vi "CollectPoint.vi"(8 "error in (no error)":errorcluster, 11 "Snake in":refnum<class "Snake.lvclass">) -> (0 "error out":errorcluster, 3 "Snake out":refnum<class "Snake.lvclass">)   [LabVIEW 2019, in "RT_Game.lvlib" / "Snake.lvclass"]
uses:
  Snake.lvclass
  Snake.lvclass/Snake.ctl
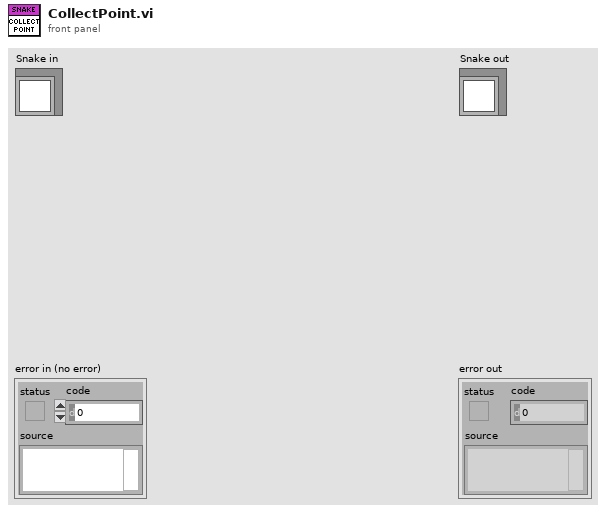
[diagram p1: front panel]
types:
  T1 = typedef "RT_Game.lvlib/Game.lvclass/Coordinate.ctl" = cluster{"x":i16, "y":i16}
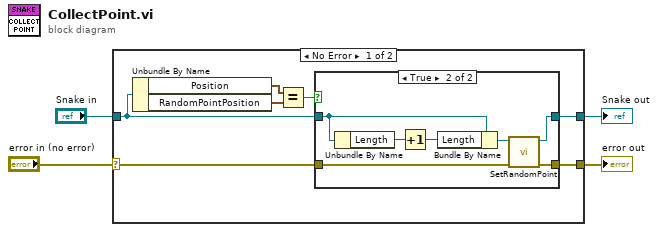
[diagram p0: block diagram]
diagram:
  n1 = case shown="No Error" "error in (no error)" {
    selector: "error in (no error)" -> [w11 w22]
    tunnel: [w8 w22] -> w3
    tunnel: [w7 w21] -> w1
    tunnel: "Snake in" -> [w6 w21]
    frame No Error {
      n2 = Unbundle By Name(w6) -> ("Position"=w9:T1, "RandomPointPosition"=w10:T1)
      n3 = Equal?(x=w9, y=w10) -> (x = y?=w5:bool)
      n4 = case shown="True" w5 {
        tunnel: w11 -> [w12 w20]
        tunnel: [w12 w19] -> w8
        tunnel: [w13 w18] -> w7
        tunnel: w6 -> [w13 w16]
        frame False {
        }
        frame True {
          n5 = Unbundle By Name(w16) -> ("Length"=w15:i16)
          n6 = Increment(x=w15) -> (x+1=w14:i16)
          n7 = Bundle By Name(cluster=w16, "Length"=w14) -> (w17:refnum<class "Snake.lvclass">)
          n8 = call "SetRandomPoint.vi"("error in (no error)"=w20, "Snake in"=w17) -> ("error out"=w19:errorcluster, "Snake out"=w18:refnum<class "Snake.lvclass">)  [unwired: 8 in]
        }
      }
    }
    frame Error {
    }
  }
  "error out" <- w3
  "Snake out" <- w1
